vi "Write.vi"(10 "U32 Array":u32[](array[numeric]), 11 "U32 Array in":refnum<class "U32 Array.lvclass">) -> (3 "U32 Array out":refnum<class "U32 Array.lvclass">)   [LabVIEW 2020, in "Data.lvlib" / "U32 Array.lvclass"]
doc: "Write U32 Array."
uses:
  U32 Array.lvclass
  U32 Array.lvclass/U32 Array.ctl
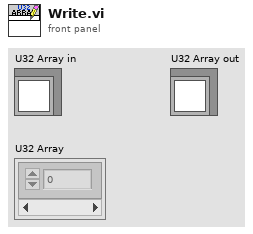
[diagram p1: front panel]
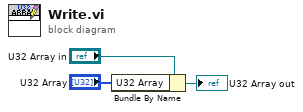
[diagram p0: block diagram]
diagram:
  n1 = Bundle By Name(cluster="U32 Array in", "U32 Array"="U32 Array") -> (→"U32 Array out":refnum<class "U32 Array.lvclass">)
